vi "ConfAndNOtProcessing.vi"(11 "Data Cluster":T1) -> (3 "result":bool)   [LabVIEW 2015, in "ISA010_module.lvlib"]
uses:
  ISA010_module.lvlib
  Module Data--cluster.ctl
  ISA010/ISA010.lvclass
  libraries/ModBUS.lvlibp/Base/Modbus.lvclass
  ISA010/Command.ctl
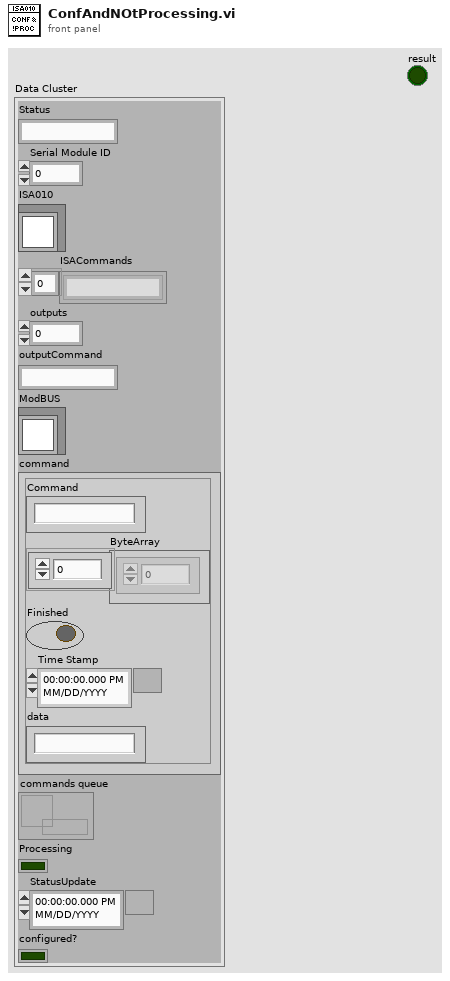
[diagram p1: front panel]
types:
  T1 = typedef "ISA010_module.lvlib/Module Data--cluster.ctl" = cluster{"Status":string, "Serial Module ID":i32, "ISA010":refnum<class "ISA010.lvclass">, "ISACommands":string[], "outputs":u16, "outputCommand":string, "ModBUS":refnum<class "Modbus.lvclass">, "command":T2, "commands queue":refnum<queue>, "Processing":bool, "StatusUpdate":timestamp, "configured?":bool}
  T2 = typedef "Command.ctl" = cluster{"Command":string, "ByteArray":u8[], "Finished":bool, "Time Stamp":timestamp, "data":string}
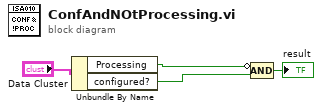
[diagram p0: block diagram]
diagram:
  n1 = Unbundle By Name("Data Cluster") -> ("Processing"=w3:bool, "configured?"=w2:bool)
  n2 = Compound Arithmetic op=AND(invert w3, w2) -> (→"result":bool)
